vi "DXF Parser.vi"(8 "error in (no error)":errorcluster, 9 "Line Trigger (SEQEND)":string="SEQEND", 11 "String in":string) -> (0 "error out":errorcluster, 3 "Output":cluster{"X":dbl[], "Y":dbl[]}[](array[cluster]))   [LabVIEW 2014]
panel:
  out "Numeric":i32
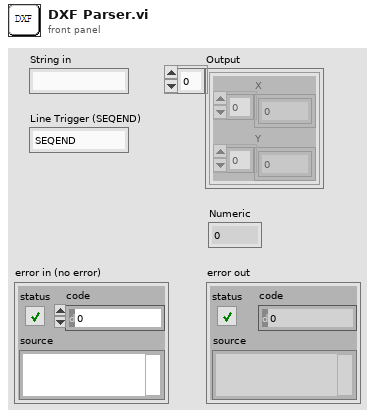
[diagram p1: front panel]
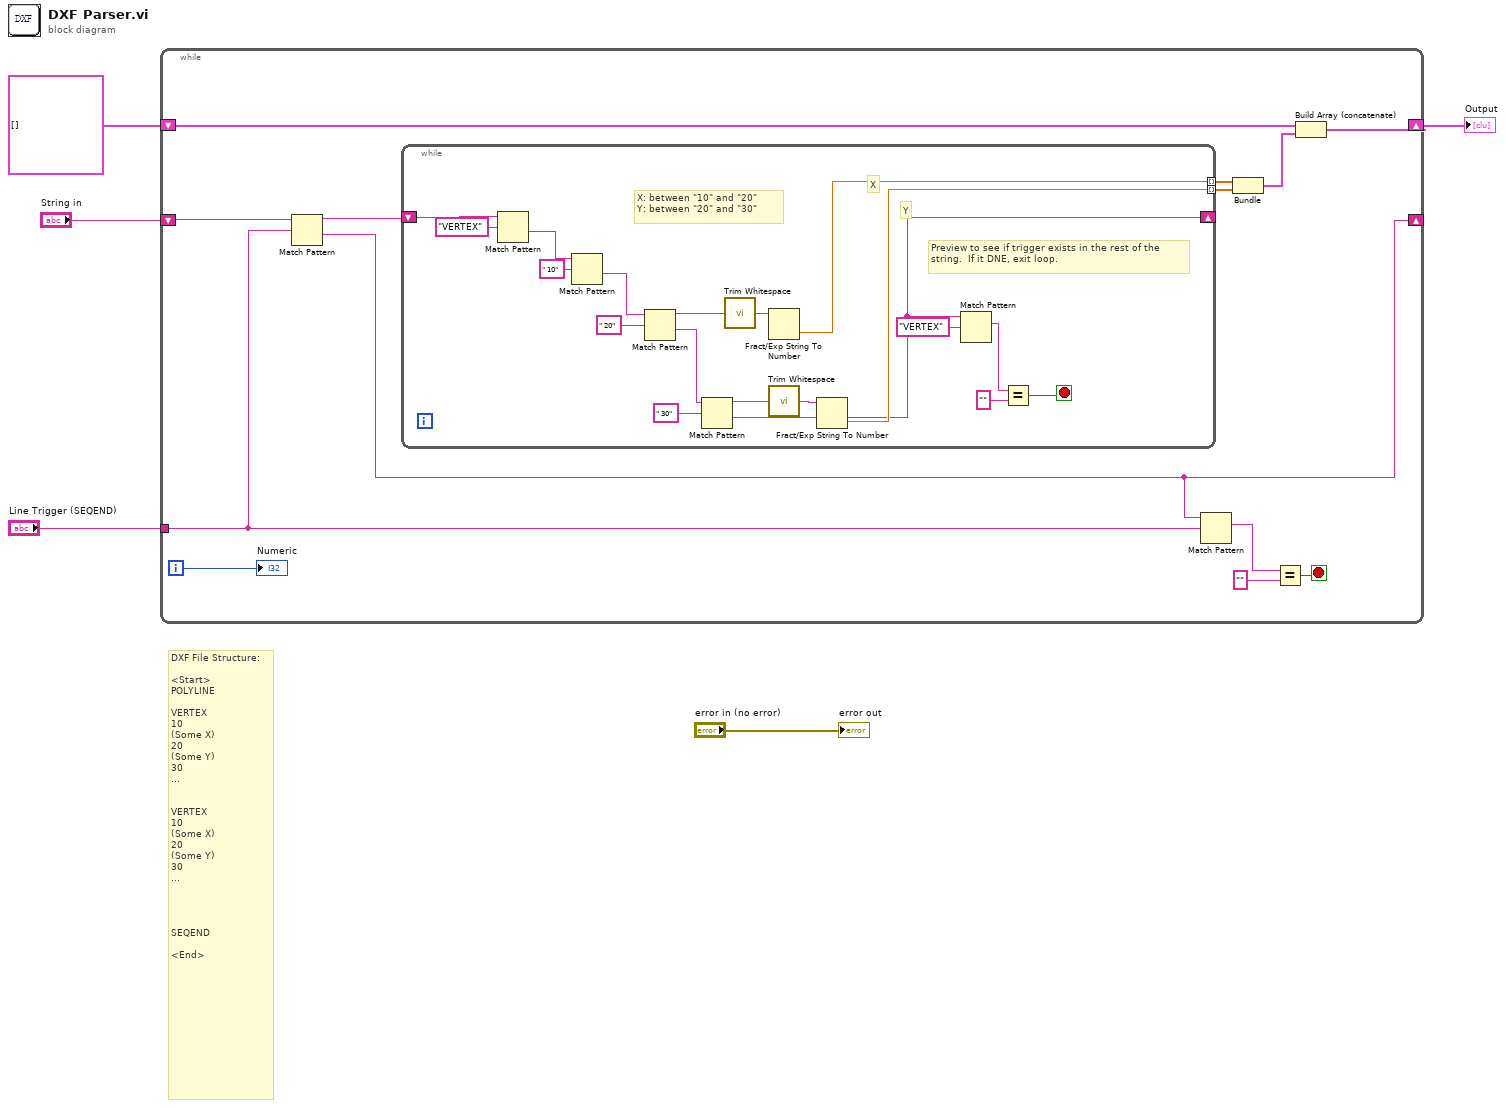
[diagram p0: block diagram]
diagram:
  # "DXF File Structure:\n\n<Start>\nPOLYLINE\n\nVERTEX\n10\n(Some X)\n20\n(Some Y)\n30\n...\n\n\nVERTEX\n10\n(Some X)\n20\n(Some Y)\n30\n...\n\n\n\n\nSEQEND\n\n<End>"
  n1 = while {
    shift-right: [w9] -> _
    shift-left: "String in" -> [w18]
    shift-right: [w6] -> w5
    shift-left: cluster{"X":dbl[], "Y":dbl[]}[] [] -> [w12]
    tunnel: "Line Trigger (SEQEND)" -> [w7]
    i -> [w11]
    stop <- w16 stop-if-true
    n2 = Match Pattern(string=w18, regular expression=w7) -> (before substring=w10:string, after substring=w9:string)  [unwired: 1 in, 2 out]
    n3 = while {
      shift-right: [w22] -> _
      shift-left: w10 -> [w26]
      tunnel: [w25] -> w15 mode=indexing
      tunnel: [w24] -> w14 mode=indexing
      stop <- w19 stop-if-true
      # "Y"
      # "X"
      # "X: between \"10\" and \"20\" \nY: between \"20\" and \"30\""
      # "Preview to see if trigger exists in the rest of the\nstring.  If it DNE, exit loop."
      n4 = Match Pattern(string=w26, regular expression="VERTEX") -> (after substring=w28:string)  [unwired: 1 in, 3 out]
      n5 = Match Pattern(string=w28, regular expression=" 10") -> (after substring=w27:string)  [unwired: 1 in, 3 out]
      n6 = Match Pattern(string=w27, regular expression=" 20") -> (before substring=w33:string, after substring=w34:string)  [unwired: 1 in, 2 out]
      n7 = Match Pattern(string=w34, regular expression=" 30") -> (before substring=w32:string, after substring=w22:string)  [unwired: 1 in, 2 out]
      n8 = call <vilib>:"Trim Whitespace.vi"("string"=w33) -> ("trimmed string"=w31:string)  [unwired: 1 in]
      n9 = Fract/Exp String To Number(string=w31) -> (number=w25:dbl)  [unwired: 3 in, 1 out]
      n10 = call <vilib>:"Trim Whitespace.vi"("string"=w32) -> ("trimmed string"=w30:string)  [unwired: 1 in]
      n11 = Fract/Exp String To Number(string=w30) -> (number=w24:dbl)  [unwired: 3 in, 1 out]
      n12 = Match Pattern(string=w22, regular expression="VERTEX") -> (match substring=w20:string)  [unwired: 1 in, 3 out]
      n13 = Equal?(x=w20, y="") -> (x = y?=w19:bool)
    }
    n14 = Match Pattern(string=w9, regular expression=w7) -> (match substring=w8:string)  [unwired: 1 in, 3 out]
    n15 = Bundle(w15, w14) -> (w13:cluster{dbl[], dbl[]})  [unwired: 1 in]
    n16 = Equal?(x=w8, y="") -> (x = y?=w16:bool)
    n17 = Build Array (concatenate)(w12, w13) -> (w6:cluster{"X":dbl[], "Y":dbl[]}[])
    "Numeric" <- w11
  }
  "Output" <- w5
  "error out" <- "error in (no error)"
